vi "TDT-Wait For Hardware.vi"(11 "error in (no error)":errorcluster) -> (15 "error out":errorcluster)   [LabVIEW 2020]
uses:
  TDT-Globals.vi
panel:
  in  "Timeout (ms)":u32=5000
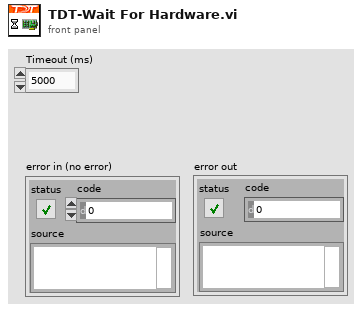
[diagram p1: front panel]
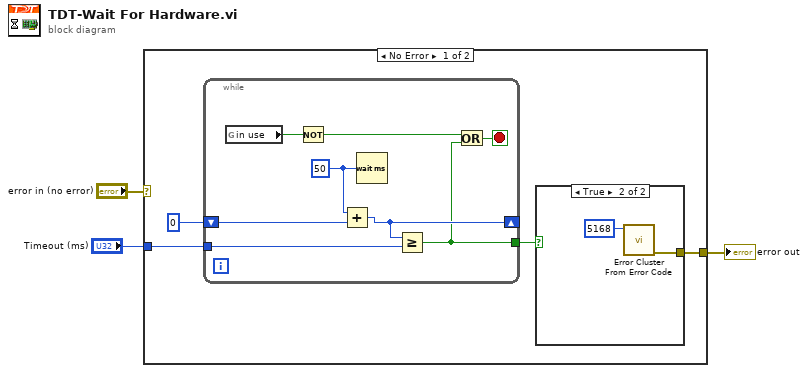
[diagram p0: block diagram]
diagram:
  n1 = case shown="No Error" "error in (no error)" {
    selector: "error in (no error)" -> [_ w18]
    tunnel: "Timeout (ms)" -> [w6 _]
    tunnel: [w4 w18] -> w2
    frame No Error {
      n2 = while {
        shift-right: [w13] -> _
        shift-left: 0 -> [w15]
        tunnel: w6 -> [w12]
        tunnel: [w10] -> w5
        stop <- w11 stop-if-true
        w14 = u32 50 ("milliseconds to wait")
        n3 = global read "TDT-Globals.vi" "in use"() -> (w9:bool)
        n4 = Not(x=w9) -> (.not. x?=w8:bool)
        n5 = Add(x=w14, y=w15) -> (x+y=w13:u32)
        n6 = Wait (ms)(milliseconds to wait=w14) -> ()  [unwired: 1 out]
        n7 = Greater Or Equal?(x=w13, y=w12) -> (x >= y?=w10:bool)
        n8 = Or(x=w8, y=w10) -> (x .or. y?=w11:bool)
      }
      n9 = case shown="True" w5 {
        tunnel: [_ w16] -> w4
        frame False {
        }
        frame True {
          n10 = call <vilib>:"Error Cluster From Error Code.vi"("error code (0)"=5168) -> ("error out"=w16:errorcluster)  [unwired: 8 in]
        }
      }
    }
    frame Error {
    }
  }
  "error out" <- w2
